vi "FTW-Actor-ClearJobs.vi"(3 "FTW Actor Instance":refnum<class "FTW-ActorInstance.lvclass">) -> (0 "FTW Actor Instance out":refnum<class "FTW-ActorInstance.lvclass">)   [LabVIEW 2015, in "FTW-ActorInstance.lvclass"]
uses:
  FTW-ActorInstance.lvclass
  FTW-ActorInstance.lvclass/FTW-ActorInstance.ctl
  JobSequencer/FTW-JobSequencer.lvclass
panel:
  # "Inputs"
  # "Outputs"
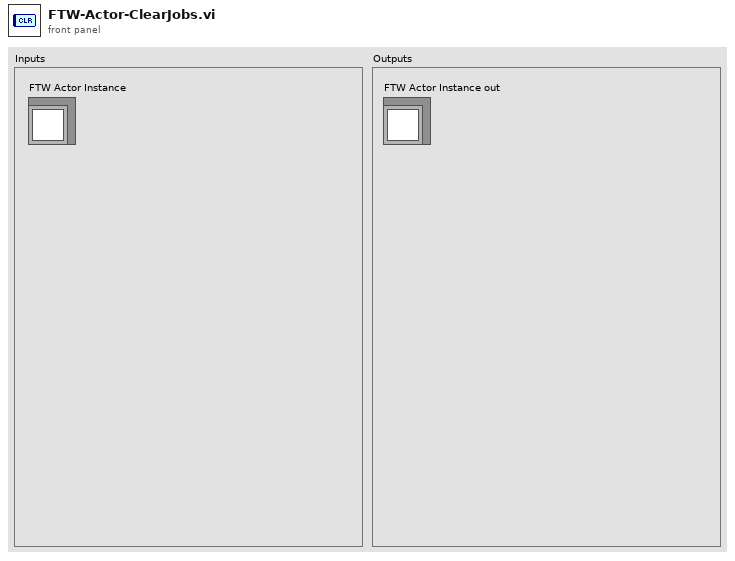
[diagram p1: front panel]
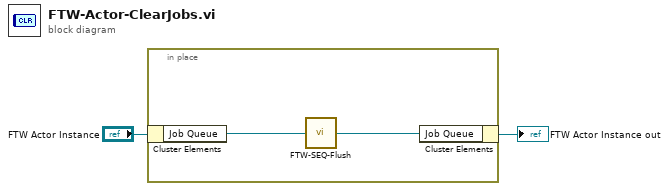
[diagram p0: block diagram]
diagram:
  n1 = in-place {
    n2 = in-place-cluster #1("FTW Actor Instance") -> ("Job Queue"=w4:refnum<class "FTW-JobSequencer.lvclass">)
    n3 = call "FTW-SEQ-Flush.vi"("FTW Job Sequencer"=w4) -> ("FTW Job Sequencer out"=w3:refnum<class "FTW-JobSequencer.lvclass">)  [unwired: 3 in]
    n4 = in-place-cluster #1("Job Queue"=w3) -> (→"FTW Actor Instance out":refnum<class "FTW-ActorInstance.lvclass">)
  }
